vi "Database File Headers.vi"() -> (4 "Rooms List Headers":string[](array[string])=["Room No", "Size", "Occupancy Status", "Occupied (Adult)", "Occupied (Children)", "Primary Guest", "Guest Contact No", "Check-In Time", "Check-out Time"], 6 "Guests History Headers":string[](array[string])=["Guest Contact No", "Primary Guest"], 8 "Room Size Details Headers":string[](array[string])=["Size", "Room Cost per Day (Rs)", "Occupancy Limit (Adult)", "Occupancy Limit (Children)"], 10 "Staffs List Headers":string[](array[string])=["Staff Name", "Designation", "Attendance"])   [LabVIEW 2023, in "File Data Manager.lvlib" / "File Data Manager.lvclass"]
uses:
  File Data Manager.lvclass
  File Data Manager.lvclass/File Data Manager.ctl
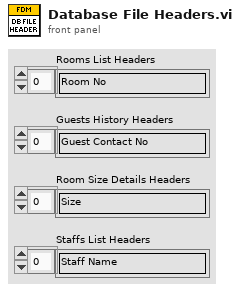
[diagram p1: front panel]
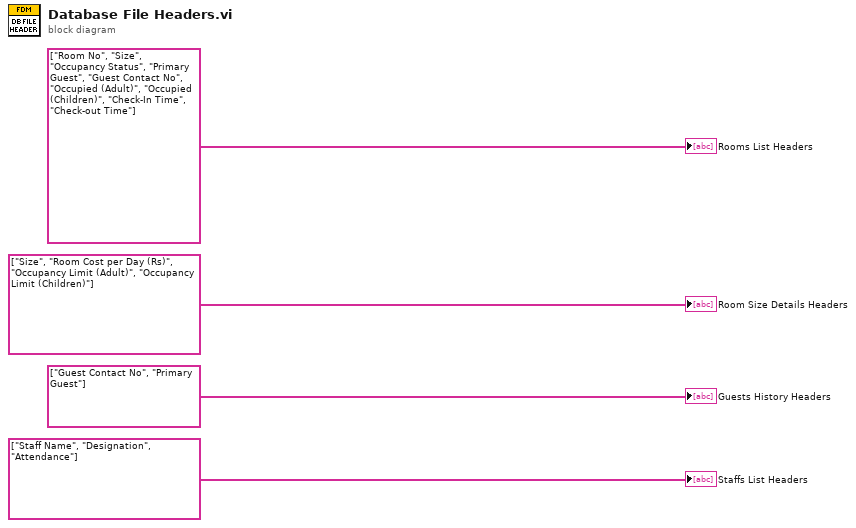
[diagram p0: block diagram]
diagram:
  "Rooms List Headers" <- string[] ["Room No", "Size", "Occupancy Status", "Primary Guest", "Guest Contact No", "Occupied (Adult)", "Occupied (Children)", "Check-In Time", "Check-out Time"] ("first row")
  "Guests History Headers" <- string[] ["Guest Contact No", "Primary Guest"] ("first row")
  "Room Size Details Headers" <- string[] ["Size", "Room Cost per Day (Rs)", "Occupancy Limit (Adult)", "Occupancy Limit (Children)"] ("first row")
  "Staffs List Headers" <- string[] ["Staff Name", "Designation", "Attendance"] ("first row")
